vi "controllerMain.vi"(8 "error in (no error)":errorcluster, 10 "UserEvents in":refnum<class "UserEvents.lvclass">, 11 "Controller in":refnum<class "Controller.lvclass">) -> (0 "error out":errorcluster, 3 "Controller out":refnum<class "Controller.lvclass">)   [LabVIEW 2013, in "Controller.lvclass"]
uses:
  Controller.lvclass
  UserEvents/UserEvents.lvclass
  StateFactory/StateFactory.lvclass
  Typedefs/StateSelector.ctl
  Model/Model/Model.lvclass
  Context/Context.lvclass
  CommandFactory/CommandFactory.lvclass
  <userlib>/Common/SerialProtocols/SerialProtocolFactory/SerialProtocolFactory/SerialProtocolFactory.lvclass
  <userlib>/Common/SerialProtocols/SerialCommunicator/SerialCommunicator.lvclass
  Model/ApplicationElements/ApplicationElements.ctl
  Model/ApplicationElements/TestMonitor/TestMonitor.lvclass
  Model/ApplicationElements/Log/TestDataLog/TestDataLog.lvclass
  Model/ApplicationElements/FlukeDMMTC/FlukeDMMTC.lvclass
  Model/ILCTC/ILCTC.lvclass
  Model/ILCSim1TC/ILCSim1TC.lvclass
  <userlib>/Common/SerialProtocols/SerialCommunicator/SerialCommunicator.lvclass/SerialCommunicator.ctl
  <userlib>/Common/Devices/FlukeDMM/FlukeDMM/FlukeDMM.lvclass/FlukeDMM.ctl
  <userlib>/Common/ILC/ILC/ILC.lvclass/ILC.ctl
  Model/Model/Model.lvclass/Model.ctl
  UserEvents/UserEvents.lvclass/UserEvents.ctl
  Context/Context.lvclass/Context.ctl
  Command/Command.lvclass
  Typedefs/AITDTTypedefs.lvlib
  <userlib>/Common/ILC/ILC/ILC.lvclass
  <userlib>/Common/Devices/FlukeDMM/FlukeDMM/FlukeDMM.lvclass
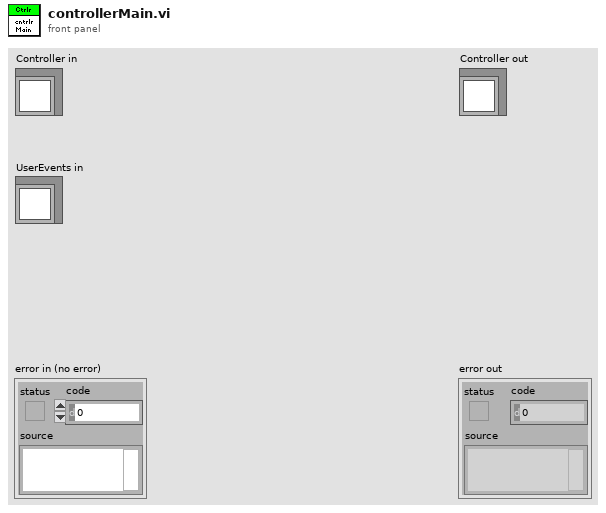
[diagram p1: front panel]
types:
  T1 = typedef "ApplicationElements.ctl" = cluster{"testMonitor":refnum<class "TestMonitor.lvclass">, "testDataLog":refnum<class "TestDataLog.lvclass">, "flukeDMMTC":refnum<class "FlukeDMMTC.lvclass">}
  T2 = typedef "AITDTTypedefs.lvlib/StateSelector.ctl" = enum16{"AwaitingSetpointAcknowledgmentState", "EndingCycleState", "FaultState", "OffState", "PausingState", "RequestingNewSetpointState", "SamplingState", "SettlingState", "SoakingState", "StabilizingState", "StandbyState", "StoppedState", "TransitioningTemperatureState"}
  T3 = typedef "AITDTTypedefs.lvlib/SubDataEvents.ctl" = cluster{"Command":refnum<user-event>}
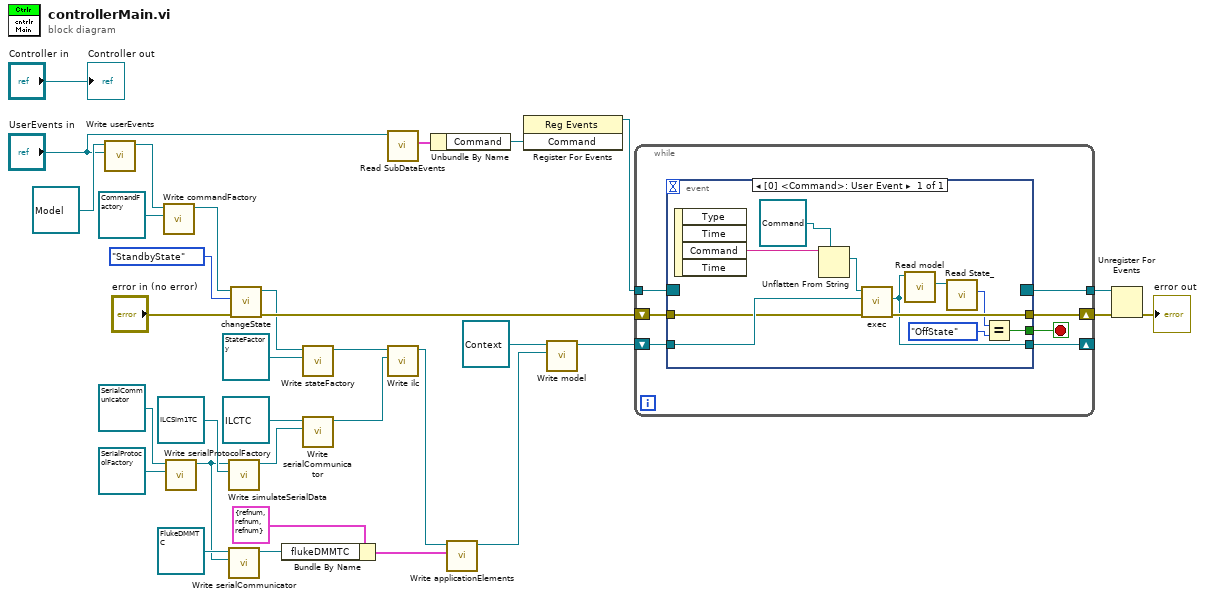
[diagram p0: block diagram]
diagram:
  n1 = call "Write userEvents.vi"("userEvents"="UserEvents in", "Model in"=refnum<class "Model.lvclass"> refnum) -> ("Model out"=w12:refnum<class "Model.lvclass">)  [unwired: 9 in]
  n2 = call "Write commandFactory.vi"("commandFactory"=refnum<class "CommandFactory.lvclass"> refnum ("CommandFactory.lvclass"), "Model in"=w12) -> ("Model out"=w10:refnum<class "Model.lvclass">)  [unwired: 9 in]
  n3 = call <userlib>:"Write serialProtocolFactory.vi"("serialProtocolFactory"=refnum<class "SerialProtocolFactory.lvclass"> refnum ("SerialCommFactory.lvclass"), "SerialCommunicator in"=refnum<class "SerialCommunicator.lvclass"> refnum ("SerialProtocols.lvlib:SerialCommunicator.lvclass")) -> ("SerialCommunicator out"=w4:refnum<class "SerialCommunicator.lvclass">)  [unwired: 9 in]
  n4 = call <userlib>:"Write simulateSerialData.vi"("simulateSerialData"=refnum<class "ILCSim1TC.lvclass"> refnum ("ILCSim1TC.lvclass"), "SerialCommunicator in"=w4) -> ("SerialCommunicator out"=w17:refnum<class "SerialCommunicator.lvclass">)  [unwired: 9 in]
  n5 = call <userlib>:"Write serialCommunicator.vi"("serialCommunicator"=w4, "FlukeDMM in"=refnum<class "FlukeDMMTC.lvclass"> refnum ("FlukeDMMTC.lvclass")) -> ("FlukeDMM out"=w1:refnum<class "FlukeDMMTC.lvclass">)  [unwired: 9 in]
  n6 = call "changeState.vi"("error in (no error)"="error in (no error)", "State:"=StateSelector."StandbyState", "Model in"=w10) -> ("error out"=w24:errorcluster, "Model out"=w8:refnum<class "Model.lvclass">)  [unwired: 7 in]
  n7 = Bundle By Name(cluster=T1 {"testMonitor"=refnum, "testDataLog"=refnum, "flukeDMMTC"=refnum} ("applicationElements"), "flukeDMMTC"=w1) -> (w2:T1)
  n8 = call "Write stateFactory.vi"("stateFactory"=refnum<class "StateFactory.lvclass"> refnum ("StateFactory.lvclass"), "Model in"=w8) -> ("Model out"=w18:refnum<class "Model.lvclass">)  [unwired: 9 in]
  n9 = call <userlib>:"Write serialCommunicator.vi"("serialCommunicator"=w17, "ILC in"=refnum<class "ILCTC.lvclass"> refnum ("ILC_TC.lvclass")) -> ("ILC out"=w19:refnum<class "ILCTC.lvclass">)  [unwired: 9 in]
  n10 = call "Read SubDataEvents.vi"("UserEvents in"="UserEvents in") -> ("SubDataEvents"=w28:T3)  [unwired: 9 in, 1 out]
  n11 = call "Write ilc.vi"("ilc"=w19, "Model in"=w18) -> ("Model out"=w16:refnum<class "Model.lvclass">)  [unwired: 9 in]
  n12 = Unbundle By Name(w28) -> ("Command"=w22:refnum<user-event>)
  n13 = call "Write applicationElements.vi"("applicationElements"=w2, "Model in"=w16) -> ("Model out"=w15:refnum<class "Model.lvclass">)  [unwired: 9 in]
  n14 = register-events(w22) -> (reference out=w27:refnum<event-registration>)  [unwired: 2 in, 1 out]
  n15 = call "Write model.vi"("Model.lvclass"=w15, "Context in"=refnum<class "Context.lvclass"> refnum ("Context.lvclass")) -> ("Context out"=w30:refnum<class "Context.lvclass">)  [unwired: 9 in]
  n16 = while {
    shift-right: [w39] -> w25
    shift-left: w24 -> [w36]
    shift-right: [w38] -> _
    shift-left: w30 -> [w40]
    tunnel: w27 -> [w35]
    tunnel: [w34] -> w26
    stop <- w37 stop-if-true
    n17 = event shown="[0] <Command>: User Event" {
      selector: w35 -> [_]
      dyn-events: [_] -> w34
      timeout: _ -> [_]
      tunnel: w40 -> [w49]
      tunnel: [w46] -> w39
      tunnel: [w45] -> w38
      tunnel: [w44] -> w37
      tunnel: w36 -> [w42]
      event User Event {
        n18 = event-data() -> ("Command"=w41:string)  [unwired: 1 in, 3 out]
        n19 = Unflatten From String(type=refnum<class "Command.lvclass"> refnum ("Command.lvclass"), binary string=w41) -> (value=w50:refnum<class "Command.lvclass">)  [unwired: 3 in, 2 out]
        n20 = call-dynamic "exec.vi"("error in (no error)"=w42, "context"=w49, "Command in"=w50) -> ("error out"=w46:errorcluster, "context 2"=w45:refnum<class "Context.lvclass">)  [unwired: 6 in, 1 out]
        n21 = call "Read model.vi"("Context in"=w45) -> ("Model.lvclass"=w48:refnum<class "Model.lvclass">)  [unwired: 9 in, 1 out]
        n22 = call "Read State_.vi"("Model in"=w48) -> ("state:"=w43:T2)  [unwired: 9 in, 1 out]
        n23 = Equal?(x=w43, y=StateSelector."OffState") -> (x = y?=w44:bool)
      }
    }
  }
  n24 = Unregister For Events(event registration refnum=w26, error in=w25) -> (error out=→"error out":errorcluster)
  "Controller out" <- "Controller in"
